vi "Init FPGA.vi"(8 "error in (no error)":errorcluster, 10 "Controller Config":T1, 11 "FPGA Ref":T3) -> (0 "error out":errorcluster, 3 "FPGA Ref Out":T3)   [LabVIEW 2019]
uses:
  Controls/FPGA_Reference.ctl
  Controls/Controller Config.ctl
  Type Defs/Controller Names.ctl
  <vilib>/FPGAPlugInAG/sbRIO-9627/niLvFpga_Reset_sbRIO-9627.vi
  <vilib>/Utility/error.llb/Error Cluster From Error Code.vi
  <vilib>/rvi/errors/niLvFpgaAdjustHostInterfaceError.vi
  <vilib>/FPGAPlugInAG/sbRIO-9627/niLvFpga_Run_sbRIO-9627.vi
  <vilib>/rvi/interface/nirviMethod/nirviMethod.xnode
  FPGA Bitfiles/LS_Durability_FPGA_9627.lvbitx
  <vilib>/rvi/interface/nirviReadWriteControl/nirviReadWriteControl.xnode
  NiFpgaLv.dll
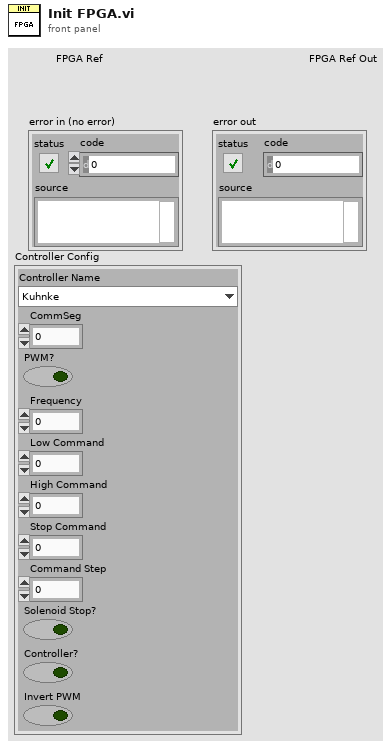
[diagram p1: front panel]
types:
  T1 = typedef "Controller Config.ctl" = cluster{"Controller Name":T2, "CommSeg":i32, "PWM?":bool, "Frequency":i32, "Low Command":dbl, "High Command":dbl, "Stop Command":dbl, "Command Step":dbl, "Solenoid Stop?":bool, "Controller?":bool, "Invert PWM":bool}
  T2 = typedef "Controller Names.ctl" = enum16{"Kuhnke", "Helbako BLDC", "Conti", "Hella BLDC OL PWM", "Hella BLDC Turbine OL PWM", "Hella BLDC Pressure", "Helbako (old)", "TI PWM", "PSA", "Hella Gas", "Hella Diesel", "8 Comm", "10 Comm", "8 Comm Hella", "10 Comm Hella", "8 Comm Omron", "10 Comm Omron", "8 Comm Nissan", "10 Comm Nissan"}
  T3 = typedef "FPGA_Reference.ctl" = refnum<k20>
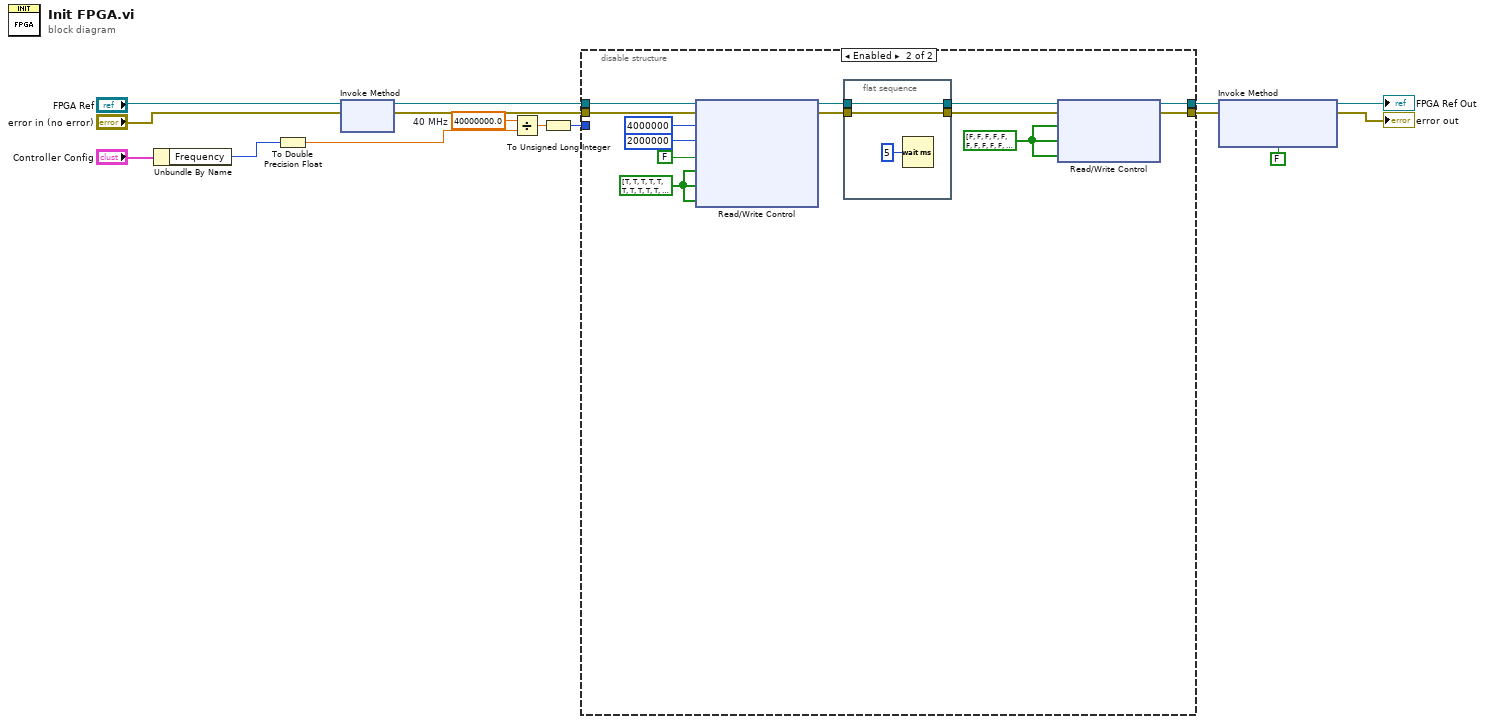
[diagram p0: block diagram]
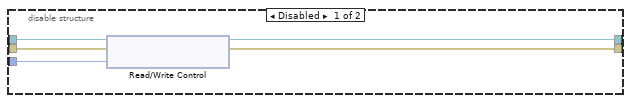
[diagram p2: hidden frame]
diagram:
  w13 = 40000000.0  # 40 MHz
  n1 = Unbundle By Name("Controller Config") -> ("Frequency"=w8:i32)
  n2 = To Double Precision Float(number=w8) -> (double precision float=w7:dbl)
  n3 = xnode "Invoke Method"("FPGA VI Reference In"="FPGA Ref", "error in"="error in (no error)") -> ("FPGA VI Reference Out"=w12:T3, "error out"=w15:errorcluster)
  n4 = Divide(x=w13, y=w7) -> (x/y=w14:dbl)
  n5 = To Unsigned Long Integer(number=w14) -> (unsigned 32bit integer=w1:u32)
  n6 = disable-structure shown="Enabled" {
    disable-tunnel: w15 -> [w20 w33]
    disable-tunnel: w12 -> [w19 w32]
    disable-tunnel: [w18 w27] -> w3
    disable-tunnel: [w17 w26] -> w2
    disable-tunnel: w1 -> [w16 _]
    frame Disabled {
      n7 = xnode "Read/Write Control"("FPGA VI Reference In"=w19, "error in"=w20, "PWM Period (Ticks)"=w16) -> ("FPGA VI Reference Out"=w18:T3, "error out"=w17:errorcluster)
    }
    frame Enabled {
      w21 = bool[] [FALSE, FALSE, FALSE, FALSE, FALSE, FALSE, FALSE, FALSE, FALSE, FALSE, FALSE, FALSE] ("Opens Resets")
      w28 = bool[] [TRUE, TRUE, TRUE, TRUE, TRUE, TRUE, TRUE, TRUE, TRUE, TRUE, TRUE, TRUE] ("Cycle Resets")
      n8 = xnode "Read/Write Control"("FPGA VI Reference In"=w32, "error in"=w33, "PWM Period (Ticks)"=u32 4000000, "Duty (Ticks)"=2000000, "Invert PWM?"=FALSE, "Cycle Resets"=w28, "Opens Resets"=w28, "Anomaly Resets"=w28) -> ("FPGA VI Reference Out"=w24:T3, "error out"=w25:errorcluster)
      n9 = flat-sequence {
        tunnel: w25 -> [w35]
        tunnel: w24 -> [w36]
        tunnel: [w36] -> w23
        tunnel: [w35] -> w22
        frame #0 {
          n10 = Wait (ms)(milliseconds to wait=u32 5) -> ()  [unwired: 1 out]
        }
      }
      n11 = xnode "Read/Write Control"("FPGA VI Reference In"=w23, "error in"=w22, "Cycle Resets"=w21, "Opens Resets"=w21, "Anomaly Resets"=w21) -> ("FPGA VI Reference Out"=w27:T3, "error out"=w26:errorcluster)
    }
  }
  n12 = xnode "Invoke Method"("FPGA VI Reference In"=w3, "error in"=w2, "Wait Until Done (F)"=FALSE) -> ("FPGA VI Reference Out"=→"FPGA Ref Out":T3, "error out"=→"error out":errorcluster)
